vi "Experimental Test.vi"() -> ()   [LabVIEW 2017]
uses:
  f5f5eb64-0c9c-4f53-a5e7-fcdb17c52b0a.vi
  Make JSON Array.vi
  Variant to JSON Text.vi
  support/Format JSON Array Text.vi
  73cd58e2-dd4a-4248-9960-3457c8e460ed.vi
  <vilib>/Utility/Data Type/NI_Data Type.lvlib
  b78c3216-ab9c-4f6e-8888-14a4e6ee3f04.vi
panel:
  out "Time/element":dbl format="%#_3p"
  out "element":string
  out "size(s)":i32
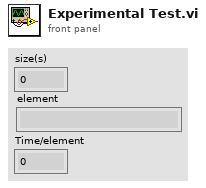
[diagram p1: front panel]
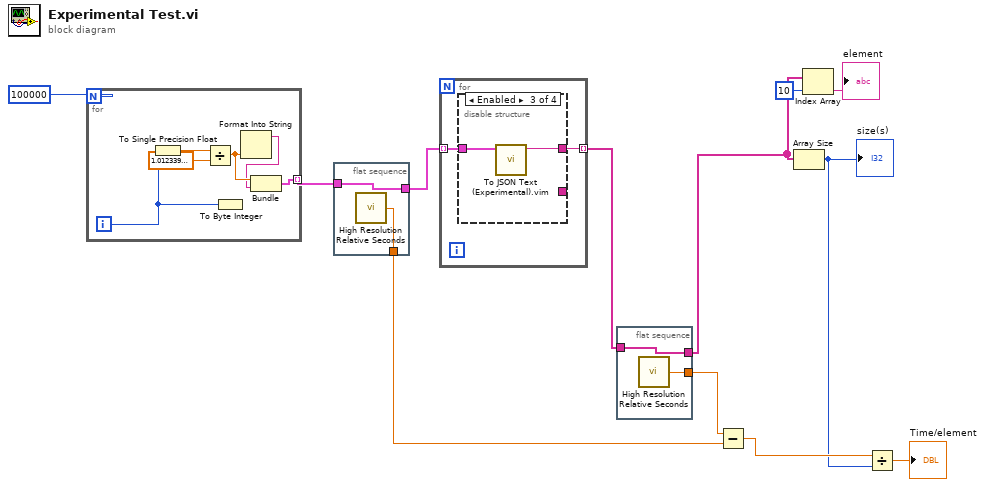
[diagram p0: block diagram]
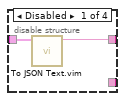
[diagram p2: hidden frame]
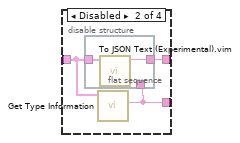
[diagram p3: hidden frame]
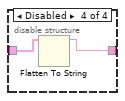
[diagram p4: hidden frame]
diagram:
  n1 = for {
    N: 100000 -> [_]
    tunnel: [w13] -> w10 mode=indexing
    i -> [w16]
    n2 = To Single Precision Float(number=w16) -> (single precision float=w18:sgl)
    n3 = Divide(x=w18, y=sgl 1.01234) -> (x/y=w15:sgl)
    n4 = To Byte Integer(number=w16) -> ()  [unwired: 1 out]
    n5 = Format Into String(w15) -> (resulting string=w14:string)  [unwired: 3 in, 1 out]
    n6 = Bundle(w15, w14) -> (w13:cluster{sgl, string})  [unwired: 1 in]
  }
  n7 = flat-sequence {
    tunnel: w10 -> [w20]
    tunnel: [w20] -> w9
    tunnel: [w19] -> w5
    frame #0 {
      n8 = call <vilib>:"High Resolution Relative Seconds.vi"() -> ("relative seconds"=w19:dbl)
    }
  }
  n9 = for {
    tunnel: w9 -> [w22] mode=indexing
    tunnel: [w21] -> w8 mode=indexing
    n10 = disable-structure shown="Enabled" {
      disable-tunnel: w22 -> [w24 w26 w30 w33]
      disable-tunnel: [w23 w27 w31 w32] -> w21
      disable-tunnel: [_ w25 _ _] -> _
      frame Disabled {
        n11 = call "To JSON Text.vim"("Anything"=w24) -> ("<JSON>"=w23:string)  [unwired: 9 in, 1 out]
      }
      frame Disabled {
        n12 = flat-sequence {
          tunnel: [w29] -> w27
          tunnel: w26 -> [w28]
          tunnel: w25 -> [_]
          frame #0 {
            n13 = call "To JSON Text (Experimental).vim"("Anything"=w28) -> ("<JSON>"=w29:string)  [unwired: 9 in, 1 out]
          }
        }
        n14 = call <vilib>:"Get Type Information.vi"("Variant"=w26) -> ("Name"=w25:string)  [unwired: 6 in, 4 out]
      }
      frame Enabled {
        n15 = call "To JSON Text (Experimental).vim"("Anything"=w30) -> ("<JSON>"=w31:string)  [unwired: 9 in, 1 out]
      }
      frame Disabled {
        n16 = Flatten To String(anything=w33) -> (data string=w32:string)  [unwired: 3 in, 2 out]
      }
    }
  }
  n17 = flat-sequence {
    tunnel: w8 -> [w35]
    tunnel: [w35] -> w7
    tunnel: [w34] -> w6
    frame #0 {
      n18 = call <vilib>:"High Resolution Relative Seconds.vi"() -> ("relative seconds"=w34:dbl)
    }
  }
  n19 = Subtract(x=w6, y=w5) -> (x-y=w4:dbl)
  n20 = Array Size(array=w7) -> (size(s)=w3:i32)
  "size(s)" <- w3
  n21 = Index Array(array=w7, index=10) -> (element=→"element":string)
  n22 = Divide(x=w4, y=w3) -> (x/y=→"Time/element":dbl)
